vi "clock_setup.vi"(0 "task in":refnum<k21>, 11 "error in":errorcluster, 12 "Dev2":bool=TRUE, 13 "Set trigger":bool=TRUE) -> (4 "task out":refnum<k21>, 15 "error out":errorcluster)   [LabVIEW 2011]
uses:
  asap/labview/initialization/globals.vi
  <vilib>/DAQmx/configure/trigger.llb/DAQmx Start Trigger (Digital Edge).vi
  Program Files (x86)/National Instruments/LabVIEW 2011/resource/objmgr/daqmx.rc
panel:
  # "Set the reference clock and triggering for a task."
  # "If true, set trigger from the usual and\ncustomary synchronization trigger."
  # "Dev2 specifies whether the task \nis on Dev1 or Dev2."
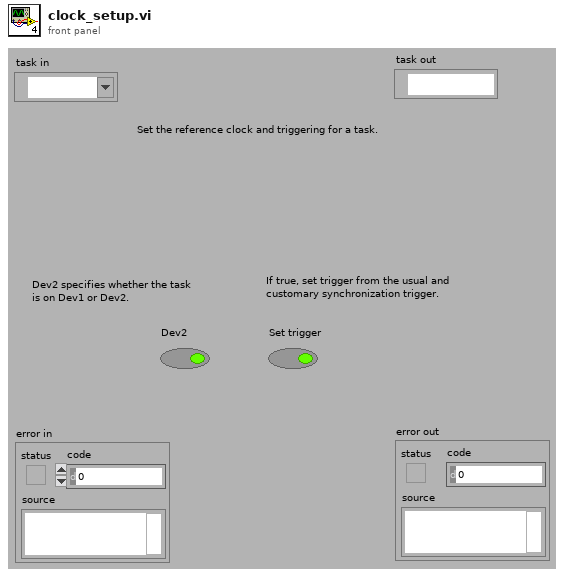
[diagram p1: front panel]
types:
  T1 = enum16{"ASAP/Trigger", "ASAP/Finder", "ASAP/Micron", "ASAP/Micron 2", "Micron 6DOF"}
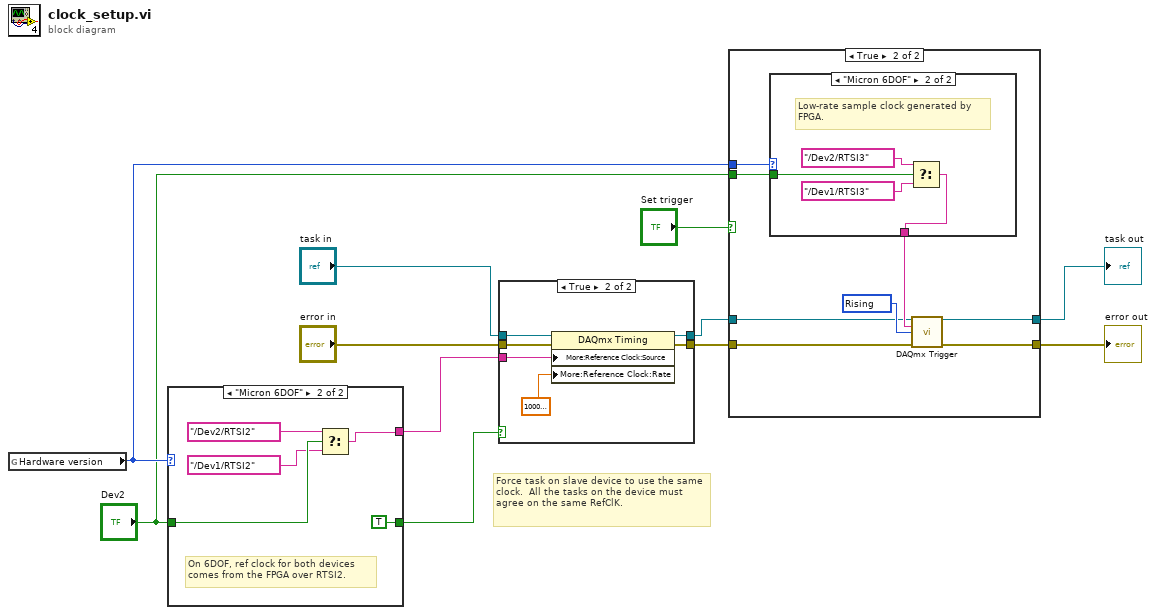
[diagram p0: block diagram]
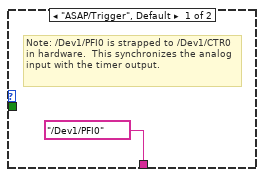
[diagram p3: hidden frame]
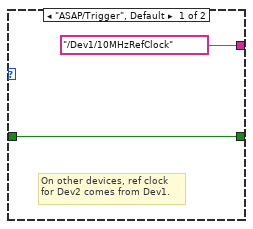
[diagram p4: hidden frame]
diagram:
  # "Force task on slave device to use the same clock.  All the tasks on the device must agree on the same RefClK."
  n1 = global read "globals.vi" "Hardware version"() -> (w2:T1)
  n2 = case shown="\"Micron 6DOF\"" w2 {
    tunnel: [tag "/Dev1/10MHzRefClock" ("RefClk.Src") w16] -> w9
    tunnel: [w12 TRUE ("Dev2")] -> w8
    tunnel: "Dev2" -> [w12 w15]
    frame "ASAP/Trigger", Default {
      # "On other devices, ref clock\nfor Dev2 comes from Dev1."
    }
    frame "Micron 6DOF" {
      # "On 6DOF, ref clock for both devices\ncomes from the FPGA over RTSI2."
      n3 = Select(t=tag "/Dev2/RTSI2" ("RefClk.Src"), s=w15, f=tag "/Dev1/RTSI2" ("RefClk.Src")) -> (s? t:f=w16:tag)
    }
  }
  n4 = case shown="True" w8 {
    tunnel: [w20 w26] -> w6
    tunnel: [w19 w25] -> w7
    tunnel: "error in" -> [w20 w24]
    tunnel: "task in" -> [w19 w23]
    tunnel: w9 -> [_ w21]
    frame False {
    }
    frame True {
      n5 = property class="DAQmx Timing"(reference=w23, error in=w24, "More:Reference Clock:Source"=w21, "More:Reference Clock:Rate"=10000000.0 ("RefClk.Rate")) -> (reference out=w25:refnum<k21>, error out=w26:errorcluster)
    }
  }
  n6 = case shown="True" "Set trigger" {
    tunnel: w7 -> [w28 w34]
    tunnel: w6 -> [w27 w33]
    tunnel: [w28 w32] -> w4
    tunnel: [w27 w31] -> w3
    tunnel: w2 -> [_ w30]
    tunnel: "Dev2" -> [_ w29]
    frame False {
    }
    frame True {
      w35 = 10280 items=["Rising"=10280, "Falling"=10171] ("edge")
      n7 = case shown="\"Micron 6DOF\"" w30 {
        tunnel: [tag "/Dev1/PFI0" ("source") w38] -> w36
        tunnel: w29 -> [_ w39]
        frame "ASAP/Trigger", Default {
          # "Note: /Dev1/PFI0 is strapped to /Dev1/CTR0 in hardware.  This synchronizes the analog input with the timer output."
        }
        frame "Micron 6DOF" {
          # "Low-rate sample clock generated by\nFPGA."
          n8 = Select(t=tag "/Dev2/RTSI3" ("RefClk.Src"), s=w39, f=tag "/Dev1/RTSI3" ("RefClk.Src")) -> (s? t:f=w38:tag)
        }
      }
      n9 = call-poly <vilib>:"DAQmx Trigger.vi"("task/channels in"=w34, "source"=w36, "edge"=w35, "error in"=w33) -> ("task out"=w32:refnum<k21>, "error out"=w31:errorcluster)  [unwired: 1 in, 9 out]
    }
  }
  "error out" <- w3
  "task out" <- w4
